vi "SOFandEOF.vi"(8 "error in (no error)":errorcluster, 11 "ISO 15693 DOWN in":refnum<class "ISO 15693 DOWN.lvclass">) -> (0 "error out":errorcluster, 3 "ISO 15693 DOWN out":refnum<class "ISO 15693 DOWN.lvclass">, 5 "frame":u8[](array[numeric]))   [LabVIEW 2019, in "ISO 15693 DOWN.lvclass"]
uses:
  ISO 15693 DOWN.lvclass
  TypeDef/Store.ctl
  ISO 15693 DOWN.lvclass/ISO 15693 DOWN.ctl
  RFID system.lvclass
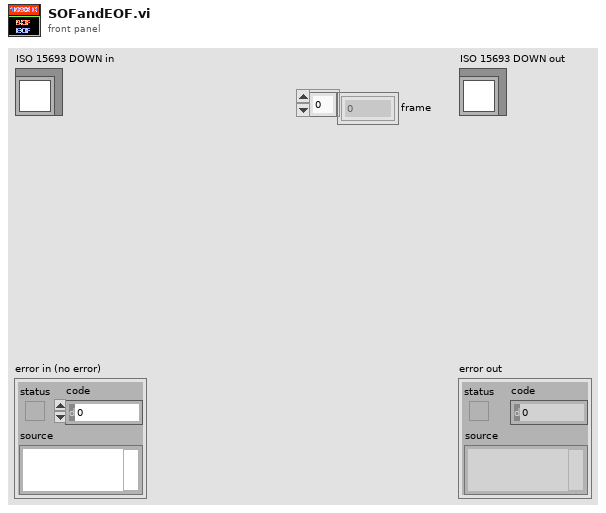
[diagram p1: front panel]
types:
  T1 = typedef "Store.ctl" = enum16{"envelope", "noise", "demSubCar", "CH_frame", "Decode", "demodulate", "in", "out", "sum", "subCarrier", "frame", "command", "encode", "modulate", "encode_UP", "modulate_up", "demod_up", "envelop_up", "sum_up", "out_up", "in_up"}
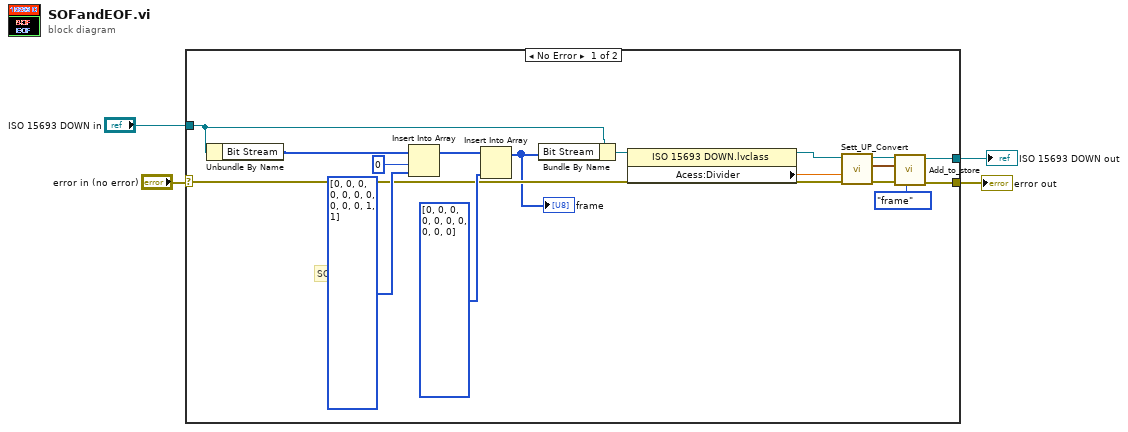
[diagram p0: block diagram]
diagram:
  n1 = case shown="No Error" "error in (no error)" {
    selector: "error in (no error)" -> [w10 w22]
    tunnel: [w12 w22] -> w3
    tunnel: "ISO 15693 DOWN in" -> [w16 w23]
    tunnel: [w9 w23] -> w1
    frame No Error {
      # "EOF"
      # "SOF"
      n2 = Unbundle By Name(w16) -> ("Bit Stream"=w17:u8[])
      n3 = Insert Into Array(array=w17, index=0, new element=u8[] [0, 0, 0, 0, 0, 0, 0, 0, 0, 0, 1, 1] ("Bit stream out (NRZ encode)")) -> (w19:u8[])
      n4 = Insert Into Array(array=w19, new element=u8[] [0, 0, 0, 0, 0, 0, 0, 0, 0, 0] ("Bit stream out (NRZ encode)")) -> (w5:u8[])  [unwired: 1 in]
      "frame" <- w5
      n5 = Bundle By Name(cluster=w16, "Bit Stream"=w5) -> (w11:refnum<class "ISO 15693 DOWN.lvclass">)
      n6 = property class="ISO 15693 DOWN.lvclass"(reference=w11) -> (reference out=w7:refnum<class "ISO 15693 DOWN.lvclass">, "Acess:Divider"=w6:dbl)  [unwired: 1 in, 1 out]
      n7 = call-dynamic "Sett_UP_Convert.vi"("error in (no error)"=w10, "Divider(1)"=w6, "ISO 15693 DOWN in"=w7) -> ("error out"=w13:errorcluster, "Waveform"=w14:waveform(dbl), "ISO 15693 DOWN out"=w15:refnum<class "ISO 15693 DOWN.lvclass">)  [unwired: 6 in]
      n8 = call "Add_to_store.vi"("Store"=Store."frame", "error in (no error)"=w13, "Waveform"=w14, "RFID system in"=w15) -> ("error out"=w12:errorcluster, "RFID system out"=w9:refnum<class "ISO 15693 DOWN.lvclass">)  [unwired: 6 in]
    }
    frame Error {
    }
  }
  "error out" <- w3
  "ISO 15693 DOWN out" <- w1
